vi "DriverStation_PanelSim_Global.vi"(0 "menu":T3=enum."set autonomous", 5 "Channel":i32, 7 "Value Set":bool, 9 "Numeric Value":dbl format="%#.4f", 11 "error in (no error)":errorcluster, 12 "String Value":string) -> (10 "Driverstation new":T1={"type"="Driverstation", "device"="", "name"="", "data"={">enabled"=FALSE, ">autonomous"=FALSE, ">test"=FALSE, ">estop"=FALSE, ">fms"=FALSE, ">ds"=FALSE, "<match_time"=0.0, ">station"="", ">game_data"=""}}, 15 "error out":errorcluster)   [LabVIEW 2019]
doc: "This is used to set and get the last motor output values. This is needed for simulation, since we cannot read these values from the hardware.\n\nThis software is licensed. Open the labview\\readme\\WPI Robotics Library Open Source License.txt file for more information."
uses:
  DS data proto.ctl
  DS proto.ctl
  DS Update Ops.ctl
panel:
  out "All Values":T1[](array[typedef])
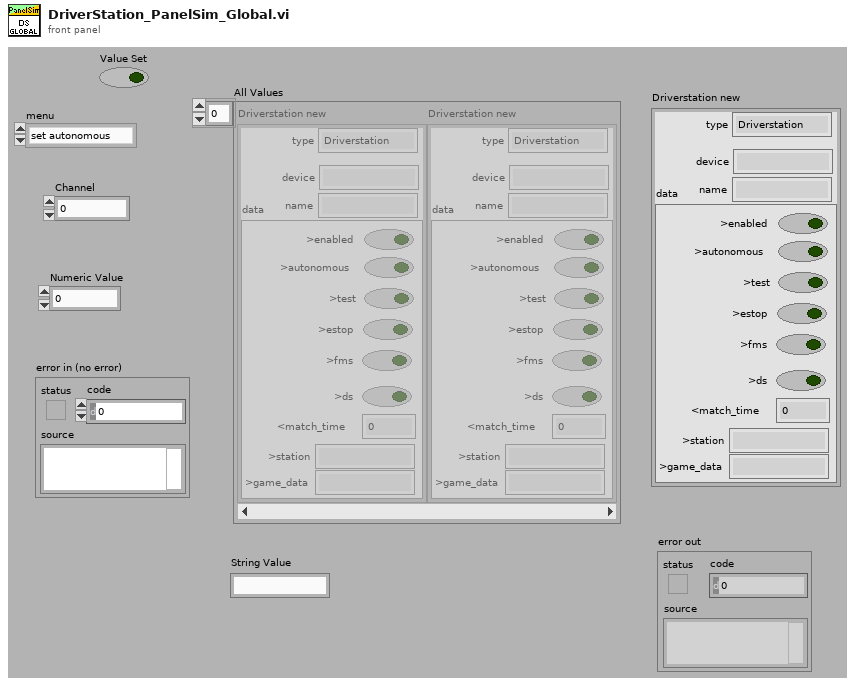
[diagram p1: front panel]
types:
  T1 = typedef "DS proto.ctl" = cluster{"type":string, "device":string, "name":string, "data":T2}
  T2 = typedef "DS data proto.ctl" = cluster{">enabled":bool, ">autonomous":bool, ">test":bool, ">estop":bool, ">fms":bool, ">ds":bool, "<match_time":dbl, ">station":string, ">game_data":string}
  T3 = typedef "DS Update Ops.ctl" = enum16{"set enabled", "set autonomous", "set test", "set estop", "set fms", "set ds", "set control word", "set match_time", "set station", "set game data", "JSON update", "set name", "get", "transmit initial", "reset"}
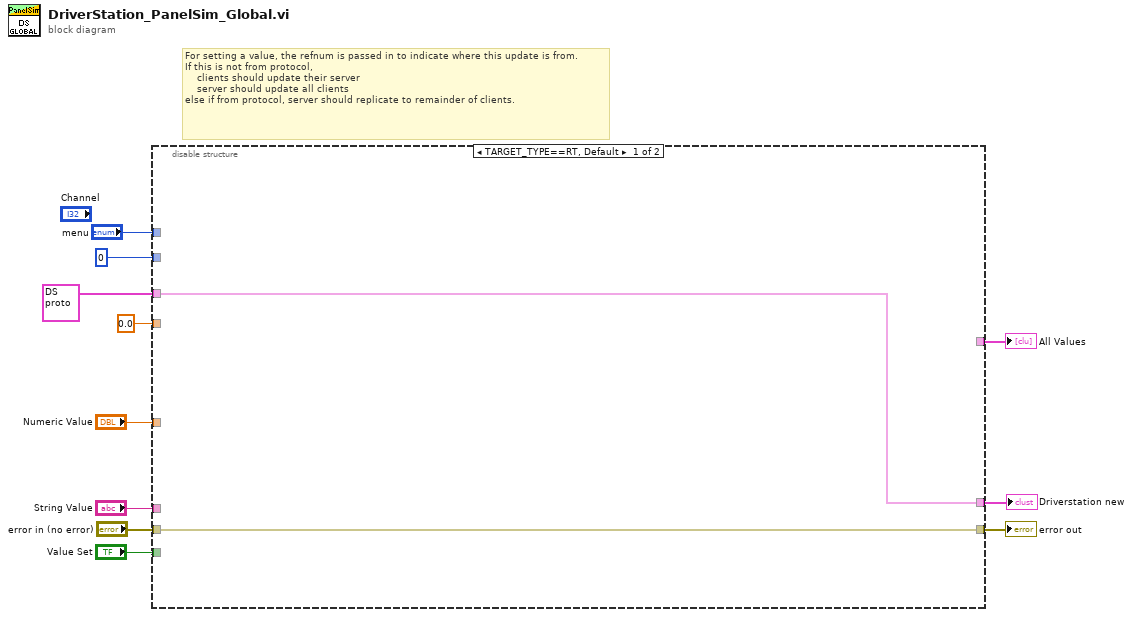
[diagram p0: block diagram]
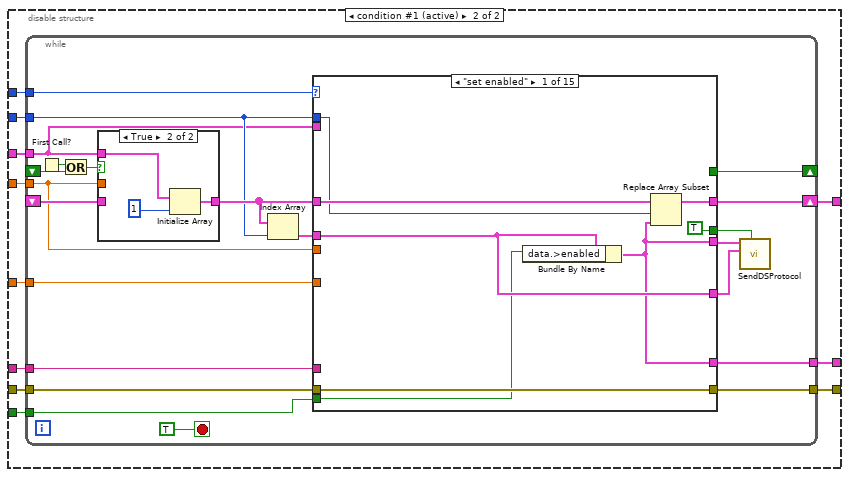
[diagram p2: hidden frame]
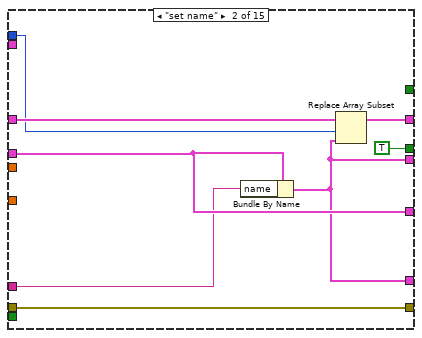
[diagram p3: hidden frame]
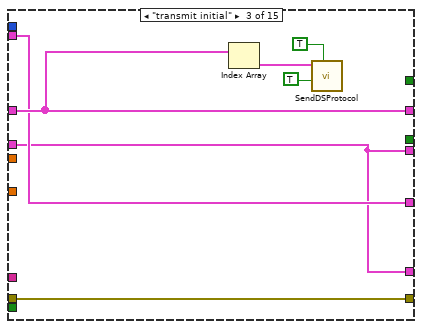
[diagram p4: hidden frame]
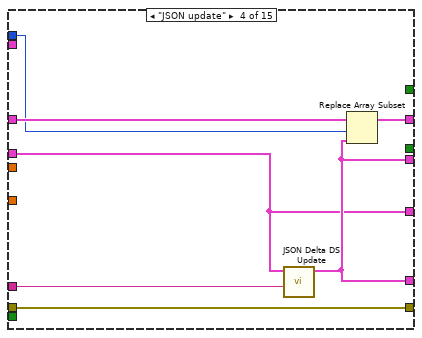
[diagram p5: hidden frame]
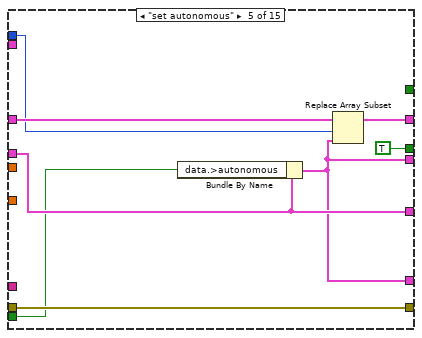
[diagram p6: hidden frame]
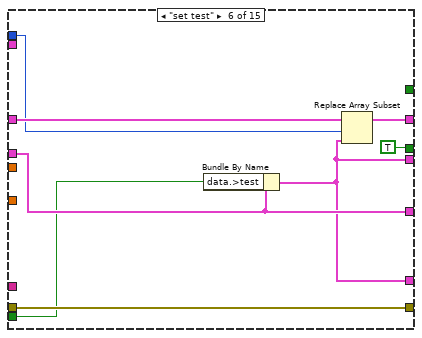
[diagram p7: hidden frame]
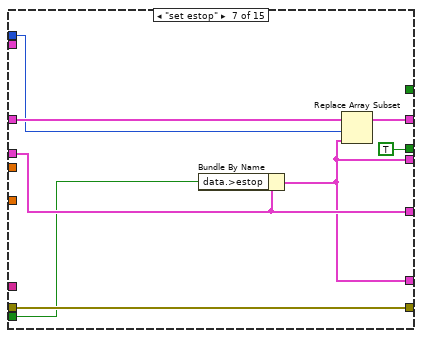
[diagram p8: hidden frame]
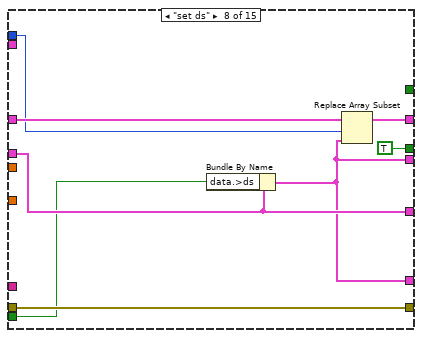
[diagram p9: hidden frame]
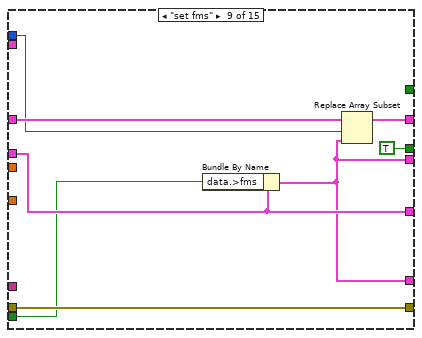
[diagram p10: hidden frame]
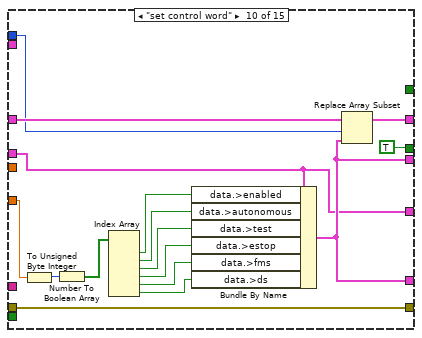
[diagram p11: hidden frame]
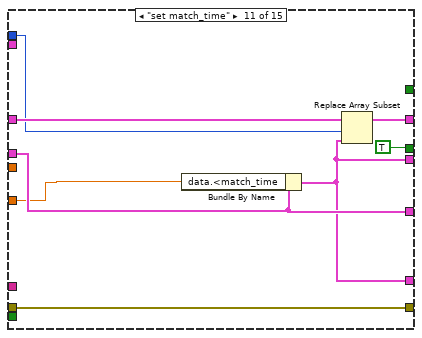
[diagram p12: hidden frame]
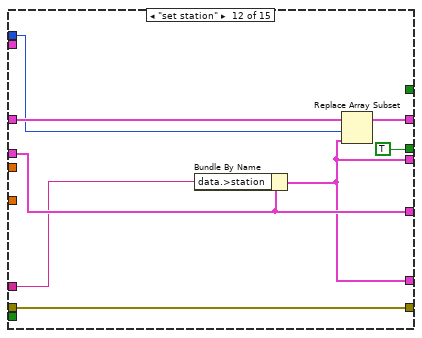
[diagram p13: hidden frame]
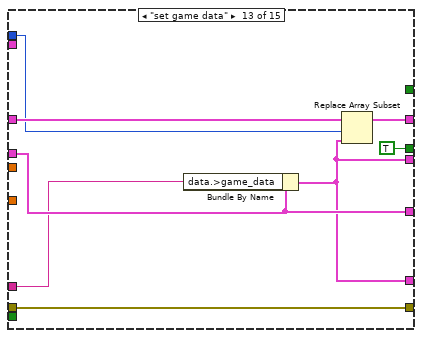
[diagram p14: hidden frame]
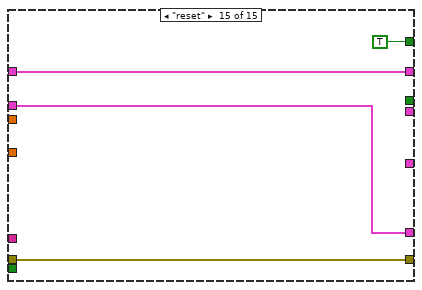
[diagram p16: hidden frame]
diagram:
  # "For setting a value, the refnum is passed in to indicate where this update is from.\nIf this is not from protocol,\n    clients should update their server\n    server should update all clients\nelse if from protocol, server should replicate to remainder of clients."
  n1 = disable-structure shown="TARGET_TYPE==RT, Default" {
    disable-tunnel: T1 {"type"="DriverStation", "device"="", "name"="", "data"={">enabled"=FALSE, ">autonomous"=FALSE, ">test"=FALSE, ">estop"=FALSE, ">fms"=FALSE, ">ds"=FALSE, "<match_time"=0.0, ">station"="", ">game_data"=""}} ("Driverstation new") -> [w12 w17]
    disable-tunnel: "menu" -> [_ w24]
    disable-tunnel: [w13 w23] -> w10
    disable-tunnel: "error in (no error)" -> [w13 w22]
    disable-tunnel: [_ w21] -> w8
    disable-tunnel: 0.0 ("Output") -> [_ w20]
    disable-tunnel: 0 -> [_ w19]
    disable-tunnel: [w12 w18] -> w6
    disable-tunnel: "String Value" -> [_ w16]
    disable-tunnel: "Numeric Value" -> [_ w15]
    disable-tunnel: "Value Set" -> [_ w14]
    frame condition #0 {
    }
    frame condition #1 (active) {
      n2 = while {
        tunnel: w22 -> [w43]
        shift-right: [w46] -> w21
        shift-left: _ -> [w39]
        tunnel: [w45] -> w18
        tunnel: w24 -> [w44]
        tunnel: [w42] -> w23
        tunnel: w19 -> [w37]
        tunnel: w20 -> [w38]
        tunnel: w17 -> [w36]
        tunnel: w16 -> [w35]
        tunnel: w15 -> [w34]
        tunnel: w14 -> [w33]
        shift-right: [w25] -> _
        shift-left: _ -> [w26]
        stop <- TRUE stop-if-true
        n3 = First Call?() -> (First Call?: T/F=w27:bool)
        n4 = Or(x=w27, y=w26) -> (x .or. y?=w28:bool)
        n5 = case shown="True" w28 {
          tunnel: [w164 w167] -> w40
          tunnel: w39 -> [w164 _]
          tunnel: w38 -> [_ _]
          tunnel: w36 -> [_ w166]
          frame False {
          }
          frame True {
            n6 = Initialize Array(w166, 1) -> (w167:T1[])
          }
        }
        n7 = Index Array(array=w40, index=w37) -> (element=w32:T1)
        n8 = case shown="\"set enabled\"" w44 {
          tunnel: [w54 w62 w68 w76 w84 w92 w100 w108 w116 w132 w140 w148 w156 w159 w163] -> w46
          tunnel: w40 -> [w52 w60 w68 w74 w82 w90 w98 w106 w114 w130 w138 w146 w154 w159 w163]
          tunnel: [w48 w56 w66 w72 w78 w86 w94 w102 w110 w127 w134 w142 w150 w157 w161] -> w45
          tunnel: [w53 w61 w69 w75 w83 w91 w99 w107 w115 w131 w139 w147 w155 w158 w162] -> w42
          tunnel: w43 -> [w53 w61 w69 w75 w83 w91 w99 w107 w115 w131 w139 w147 w155 w158 w162]
          tunnel: w37 -> [w50 w58 _ w73 w80 w88 w96 w104 w112 w128 w136 w144 w152 _ _]
          tunnel: w38 -> [_ _ _ _ _ _ _ _ _ _ _ _ _ _ _]
          tunnel: [w48 w56 w66 w72 w78 w86 w94 w102 w110 w127 w134 w142 w150 _ _] -> w30
          tunnel: [w49 w57 w67 w70 w79 w87 w95 w103 w111 w122 w135 w143 w151 _ _] -> w31
          tunnel: [TRUE TRUE _ _ TRUE TRUE TRUE TRUE TRUE TRUE TRUE TRUE TRUE _ _] -> w29
          tunnel: w32 -> [w49 w57 w66 w70 w79 w87 w95 w103 w111 w122 w135 w143 w151 w157 w161]
          tunnel: w36 -> [_ _ w67 _ _ _ _ _ _ _ _ _ _ _ _]
          tunnel: w35 -> [_ w55 _ w71 _ _ _ _ _ _ _ w141 w149 _ _]
          tunnel: w34 -> [_ _ _ _ _ _ _ _ _ w126 w133 _ _ _ _]
          tunnel: w33 -> [w47 _ _ _ w77 w85 w93 w101 w109 _ _ _ _ _ _]
          tunnel: [_ _ _ _ _ _ _ _ _ _ _ _ _ _ TRUE] -> w25
          frame "set enabled" {
            n9 = Bundle By Name(cluster=w49, "data.>enabled"=w47) -> (w48:T1)
            n10 = Replace Array Subset(array=w52, new element=w48, index=w50) -> (w54:T1[])
          }
          frame "set name" {
            n11 = Bundle By Name(cluster=w57, "name"=w55) -> (w56:T1)
            n12 = Replace Array Subset(array=w60, new element=w56, index=w58) -> (w62:T1[])
          }
          frame "transmit initial" {
            n13 = Index Array(array=w68) -> (element=w63:T1)  [unwired: 1 in]
            n14 = call "SendDSProtocol.vi"("Send"=TRUE, "Initialize"=TRUE, "DS new"=w63) -> ()  [unwired: 9 in]
          }
          frame "JSON update" {
            n15 = call "JSON Delta DS Update.vi"("Delta JSON"=w71, "input"=w70) -> ("output"=w72:T1)  [unwired: 8 in, 1 out]
            n16 = Replace Array Subset(array=w74, new element=w72, index=w73) -> (w76:T1[])
          }
          frame "set autonomous" {
            n17 = Bundle By Name(cluster=w79, "data.>autonomous"=w77) -> (w78:T1)
            n18 = Replace Array Subset(array=w82, new element=w78, index=w80) -> (w84:T1[])
          }
          frame "set test" {
            n19 = Bundle By Name(cluster=w87, "data.>test"=w85) -> (w86:T1)
            n20 = Replace Array Subset(array=w90, new element=w86, index=w88) -> (w92:T1[])
          }
          frame "set estop" {
            n21 = Bundle By Name(cluster=w95, "data.>estop"=w93) -> (w94:T1)
            n22 = Replace Array Subset(array=w98, new element=w94, index=w96) -> (w100:T1[])
          }
          frame "set ds" {
            n23 = Bundle By Name(cluster=w103, "data.>ds"=w101) -> (w102:T1)
            n24 = Replace Array Subset(array=w106, new element=w102, index=w104) -> (w108:T1[])
          }
          frame "set fms" {
            n25 = Bundle By Name(cluster=w111, "data.>fms"=w109) -> (w110:T1)
            n26 = Replace Array Subset(array=w114, new element=w110, index=w112) -> (w116:T1[])
          }
          frame "set control word" {
            n27 = To Unsigned Byte Integer(number=w126) -> (unsigned 8bit integer=w125:u8)
            n28 = Number To Boolean Array(number=w125) -> (Boolean array=w124:bool[])
            n29 = Index Array(array=w124) -> (element #1=w123:bool, element #2=w121:bool, element #3=w120:bool, element #4=w119:bool, element #5=w118:bool, element #6=w117:bool)  [unwired: 6 in]
            n30 = Bundle By Name(cluster=w122, "data.>enabled"=w123, "data.>autonomous"=w121, "data.>test"=w120, "data.>estop"=w119, "data.>fms"=w118, "data.>ds"=w117) -> (w127:T1)
            n31 = Replace Array Subset(array=w130, new element=w127, index=w128) -> (w132:T1[])
          }
          frame "set match_time" {
            n32 = Bundle By Name(cluster=w135, "data.<match_time"=w133) -> (w134:T1)
            n33 = Replace Array Subset(array=w138, new element=w134, index=w136) -> (w140:T1[])
          }
          frame "set station" {
            n34 = Bundle By Name(cluster=w143, "data.>station"=w141) -> (w142:T1)
            n35 = Replace Array Subset(array=w146, new element=w142, index=w144) -> (w148:T1[])
          }
          frame "set game data" {
            n36 = Bundle By Name(cluster=w151, "data.>game_data"=w149) -> (w150:T1)
            n37 = Replace Array Subset(array=w154, new element=w150, index=w152) -> (w156:T1[])
          }
          frame "get" {
          }
          frame "reset" {
          }
        }
        n38 = call "SendDSProtocol.vi"("Send"=w29, "DS old"=w31, "DS new"=w30) -> ()  [unwired: 9 in]
      }
    }
  }
  "error out" <- w10
  "All Values" <- w8
  "Driverstation new" <- w6
